vi "con_strs.vi"(11 "输出簇":T1) -> (3 "连接的字符串":string)   [LabVIEW 2012]
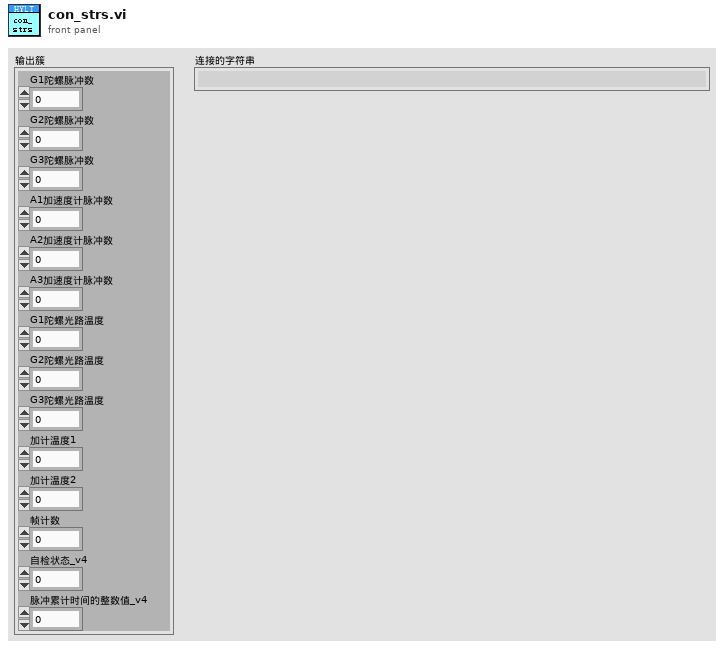
[diagram p1: front panel]
types:
  T1 = cluster{"G1陀螺脉冲数":i32, "G2陀螺脉冲数":i32, "G3陀螺脉冲数":i32, "A1加速度计脉冲数":i32, "A2加速度计脉冲数":i32, "A3加速度计脉冲数":i32, "G1陀螺光路温度":u8, "G2陀螺光路温度":u8, "G3陀螺光路温度":u8, "加计温度1":u8, "加计温度2":u8, "帧计数":u8, "自检状态_v4":u8, "脉冲累计时间的整数值_v4":u16}
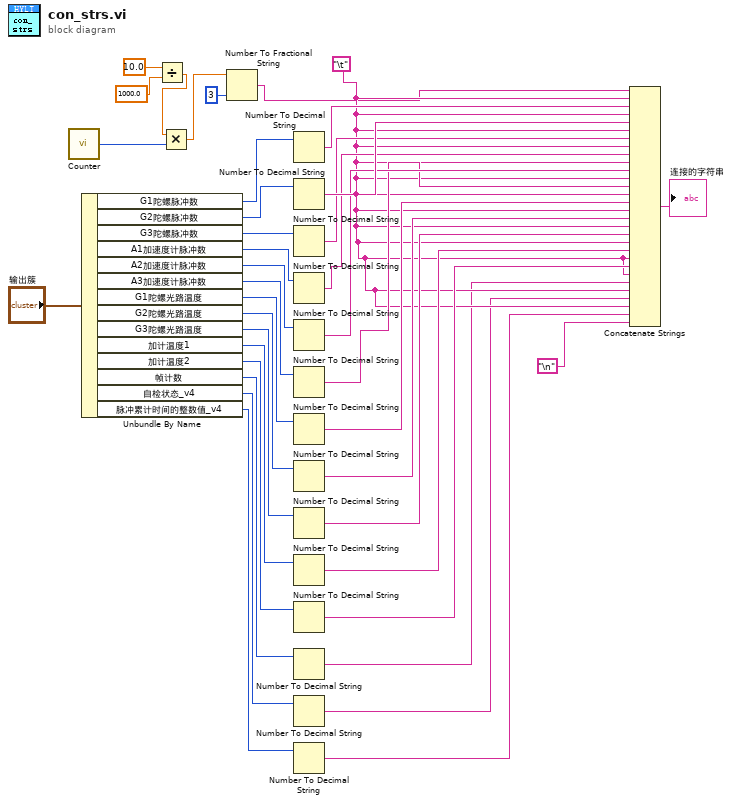
[diagram p0: block diagram]
diagram:
  w13 = "\t"
  n1 = call "Counter.vi"() -> ("Counter"=w2:u64)  [unwired: 1 in]
  n2 = Unbundle By Name("输出簇") -> ("G1陀螺脉冲数"=w38:i32, "G2陀螺脉冲数"=w37:i32, "G3陀螺脉冲数"=w36:i32, "A1加速度计脉冲数"=w35:i32, "A2加速度计脉冲数"=w34:i32, "A3加速度计脉冲数"=w33:i32, "G1陀螺光路温度"=w32:u8, "G2陀螺光路温度"=w31:u8, "G3陀螺光路温度"=w30:u8, "加计温度1"=w29:u8, "加计温度2"=w28:u8, "帧计数"=w27:u8, "自检状态_v4"=w26:u8, "脉冲累计时间的整数值_v4"=w25:u16)
  n3 = Divide(x=sgl 10.0, y=sgl 1000.0) -> (x/y=w3:sgl)
  n4 = Multiply(x=w3, y=w2) -> (x*y=w1:sgl)
  n5 = Number To Fractional String(number=w1, precision (6)=i16 3 ("精度(6)")) -> (F-format string=w4:string)  [unwired: 2 in]
  n6 = Number To Decimal String(number=w38) -> (decimal integer string=w24:string)  [unwired: 1 in]
  n7 = Number To Decimal String(number=w37) -> (decimal integer string=w23:string)  [unwired: 1 in]
  n8 = Number To Decimal String(number=w36) -> (decimal integer string=w22:string)  [unwired: 1 in]
  n9 = Number To Decimal String(number=w35) -> (decimal integer string=w21:string)  [unwired: 1 in]
  n10 = Number To Decimal String(number=w34) -> (decimal integer string=w20:string)  [unwired: 1 in]
  n11 = Number To Decimal String(number=w33) -> (decimal integer string=w19:string)  [unwired: 1 in]
  n12 = Number To Decimal String(number=w32) -> (decimal integer string=w18:string)  [unwired: 1 in]
  n13 = Number To Decimal String(number=w31) -> (decimal integer string=w17:string)  [unwired: 1 in]
  n14 = Number To Decimal String(number=w30) -> (decimal integer string=w16:string)  [unwired: 1 in]
  n15 = Number To Decimal String(number=w29) -> (decimal integer string=w15:string)  [unwired: 1 in]
  n16 = Number To Decimal String(number=w28) -> (decimal integer string=w14:string)  [unwired: 1 in]
  n17 = Number To Decimal String(number=w27) -> (decimal integer string=w12:string)  [unwired: 1 in]
  n18 = Number To Decimal String(number=w26) -> (decimal integer string=w11:string)  [unwired: 1 in]
  n19 = Number To Decimal String(number=w25) -> (decimal integer string=w10:string)  [unwired: 1 in]
  n20 = Concatenate Strings(w4, w13, w24, w13, w23, w13, w22, w13, w21, w13, w20, w13, w19, w13, w18, w13, w17, w13, w16, w13, w15, w13, w14, w13, w12, w13, w11, w13, w10, "\n") -> (→"连接的字符串":string)
